vi "CorrectClockLag.vi"(8 "error in (no error)":errorcluster, 10 "data (time, freq, amplitude, phase)":dbl[][](array[numeric]) format="%#.7g", 11 "SpinCore in":refnum<class "SpinCore.lvclass">) -> (0 "error out":errorcluster, 2 "data (time, freq, amplitude, phase)":dbl[][](array[numeric]) format="%_9g", 3 "SpinCore out":refnum<class "SpinCore.lvclass">)   [LabVIEW 2011, in "Hardware.lvlib" / "Channels.lvlib" / "SpinCore.lvclass"]
uses:
  SpinCore.lvclass
  SpinCore.lvclass/SpinCore.ctl
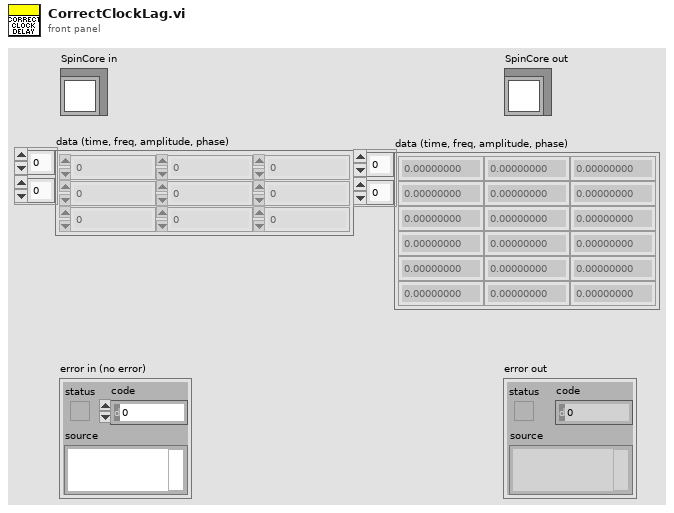
[diagram p1: front panel]
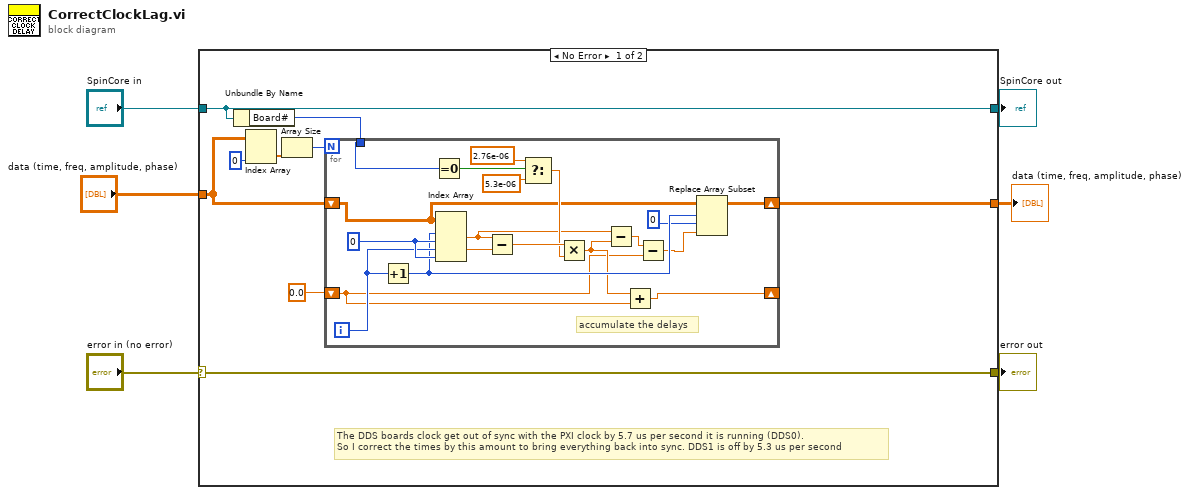
[diagram p0: block diagram]
diagram:
  n1 = case shown="No Error" "error in (no error)" {
    selector: "error in (no error)" -> [w15 w36]
    tunnel: [w15 w36] -> w5
    tunnel: [w10 w35] -> w3
    tunnel: "SpinCore in" -> [w10 w35]
    tunnel: "data (time, freq, amplitude, phase)" -> [w11 _]
    tunnel: [w8 _] -> w1
    frame No Error {
      # "The DDS boards clock get out of sync with the PXI clock by 5.7 us per second it is running (DDS0).\nSo I correct the times by this amount to bring everything back into sync. DDS1 is off by 5.3 us per second"
      n2 = Unbundle By Name(w10) -> ("Board#"=w9:i32)
      n3 = Index Array(array=w11, index (col)=0) -> (element=w12:dbl[])  [unwired: 1 in]
      n4 = Array Size(array=w12) -> (size(s)=w13:i32)
      n5 = for {
        N: w13 -> [_]
        tunnel: w9 -> [w30]
        shift-right: [w21] -> w8
        shift-left: w11 -> [w24]
        shift-right: [w16] -> _
        shift-left: 0.0 -> [w17]
        i -> [w32]
        w33 = 0
        # "accumulate the delays"
        n6 = Increment(x=w32) -> (x+1=w23:i32)
        n7 = Equal To 0?(x=w30) -> (x = 0?=w29:bool)
        n8 = Index Array(array=w24, index (row) #1=w23, index (col) #1=w33, index (row) #2=w32, index (col) #2=w33) -> (element #1=w25:dbl, element #2=w34:dbl)
        n9 = Subtract(x=w25, y=w34) -> (x-y=w31:dbl)
        n10 = Select(t=2.76e-06, s=w29, f=5.3e-06) -> (s? t:f=w26:dbl)
        n11 = Multiply(x=w31, y=w26) -> (x*y=w18:dbl)
        n12 = Subtract(x=w25, y=w18) -> (x-y=w20:dbl)
        n13 = Add(x=w18, y=w17) -> (x+y=w16:dbl)
        n14 = Subtract(x=w20, y=w17) -> (x-y=w19:dbl)
        n15 = Replace Array Subset(array=w24, new element=w19, index (row)=w23, index (col)=0) -> (w21:dbl[][])
      }
    }
    frame Error {
    }
  }
  "error out" <- w5
  "SpinCore out" <- w3
  "data (time, freq, amplitude, phase)" <- w1
